vi "SetCurrentScreen.vi"(8 "error in (no error)":errorcluster, 11 "Pong in":refnum<class "Pong.lvclass">) -> (0 "error out":errorcluster, 3 "Pong out":refnum<class "Pong.lvclass">)   [LabVIEW 2019, in "RT_Game.lvlib" / "Pong.lvclass"]
uses:
  Pong.lvclass
  Game/Game.lvclass
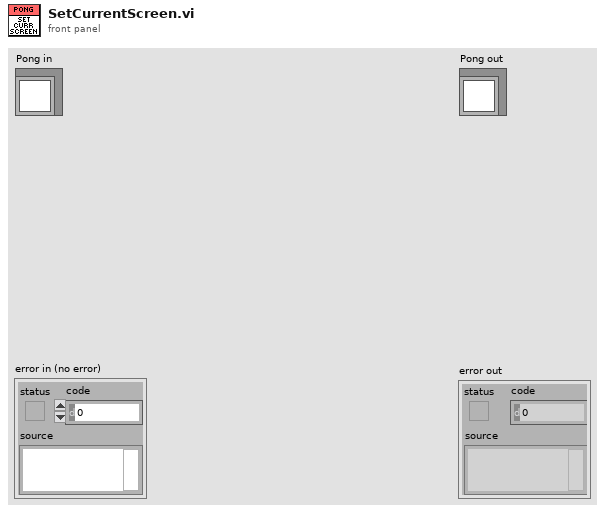
[diagram p1: front panel]
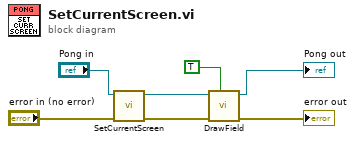
[diagram p0: block diagram]
diagram:
  n1 = call-parent "SetCurrentScreen.vi"("error in (no error)"="error in (no error)", "Game in"="Pong in") -> ("error out"=w7:errorcluster, "Game out"=w3:refnum<class "Pong.lvclass">)  [unwired: 8 in]
  n2 = call "DrawField.vi"("ForceDraw?"=TRUE, "error in (no error)"=w7, "Pong in"=w3) -> ("error out"=→"error out":errorcluster, "Pong out"=→"Pong out":refnum<class "Pong.lvclass">)  [unwired: 7 in]
